vi "FPGA Write By Name - U16.vi"(8 "error in (no error)":errorcluster, 9 "Value":u16, 10 "Control":string, 11 "FPGA Session In":refnum<class "FPGA Interface Base.lvclass">) -> (0 "error out":errorcluster, 3 "FPGA Session Out":refnum<class "FPGA Interface Base.lvclass">)   [LabVIEW 2010, in "FPGA Interface Base.lvclass"]
doc: "Writes an unsigned 16-bit integer value to a given control or indicator."
uses:
  <userlib>/_FPGA Interface Advanced Tools/FPGA Interface Base/FPGA Interface Base.lvclass
  <vilib>/rvi/DataTransferAndStorage/Container/Common/niFpgaDataTypeControl.ctl
  <userlib>/_FPGA Interface Advanced Tools/FPGA Interface Base/FPGA Interface Base.lvclass/FPGA Interface Base.ctl
  <vilib>/Utility/error.llb/Error Cluster From Error Code.vi
  <userlib>/_FPGA Interface Advanced Tools/FPGA Interface Base/Accessors/FPGA Read Session.vi
  <userlib>/_FPGA Interface Advanced Tools/FPGA Interface Wrapper/FPGA Interface Wrapper.lvlib
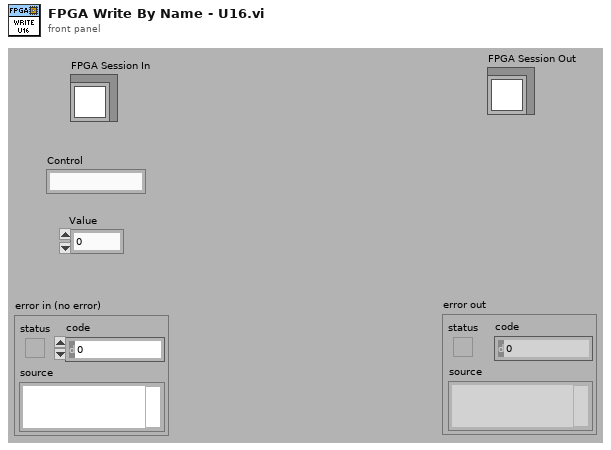
[diagram p1: front panel]
types:
  T1 = typedef "niFpgaDataTypeControl.ctl" = enum32{"Boolean", "I8", "I16", "I32", "I64", "U8", "U16", "U32", "U64", "FXP", "CustomControl"}
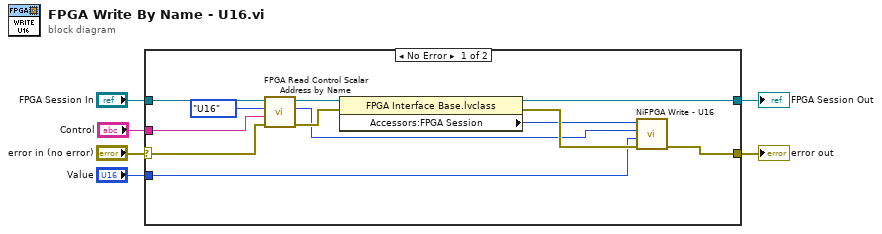
[diagram p0: block diagram]
diagram:
  n1 = case shown="No Error" "error in (no error)" {
    selector: "error in (no error)" -> [w13 w20]
    tunnel: [w15 w20] -> w1
    tunnel: [w16 w19] -> w2
    tunnel: "FPGA Session In" -> [w9 w19]
    tunnel: "Control" -> [w7 _]
    tunnel: "Value" -> [w14 _]
    frame No Error {
      n2 = call <userlib>:"FPGA Read Control Scalar Address by Name.vi"("error in (no error)"=w13, "Name"=w7, "Data Type"=niFpgaDataTypeControl."U16", "FPGA Interface Base in"=w9) -> ("error out"=w12:errorcluster, "Address"=w11:u32, "FPGA Interface Base out"=w10:refnum<class "FPGA Interface Base.lvclass">)  [unwired: 4 in, 1 out]
      n3 = property class="FPGA Interface Base.lvclass"(reference=w10, error in=w12) -> (reference out=w16:refnum<class "FPGA Interface Base.lvclass">, error out=w18:errorcluster, "Accessors:FPGA Session"=w17:u32)
      n4 = call <userlib>:"NiFPGA Write - U16.vi"("error in (no error)"=w18, "Value"=w14, "Control"=w11, "Session"=w17) -> ("error out"=w15:errorcluster)  [unwired: 6 in, 1 out]
    }
    frame Error {
    }
  }
  "error out" <- w1
  "FPGA Session Out" <- w2
